vi "Serialize.vi"(0 "object in":refnum<class "Serializer.lvclass">, 2 "outputs":variant[](array[variant]), 5 "error in (no error)":errorcluster) -> (14 "object out":refnum<class "Serializer.lvclass">, 16 "JSON":string, 19 "error out":errorcluster)   [LabVIEW 2018, in "Serializer.lvclass"]
doc: "Serialize the output data to string in a format determined by the child class."
uses:
  Serializer.lvclass
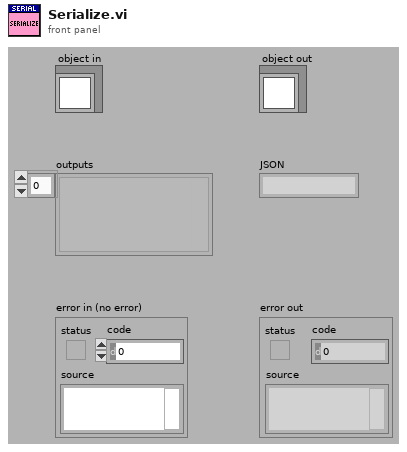
[diagram p1: front panel]
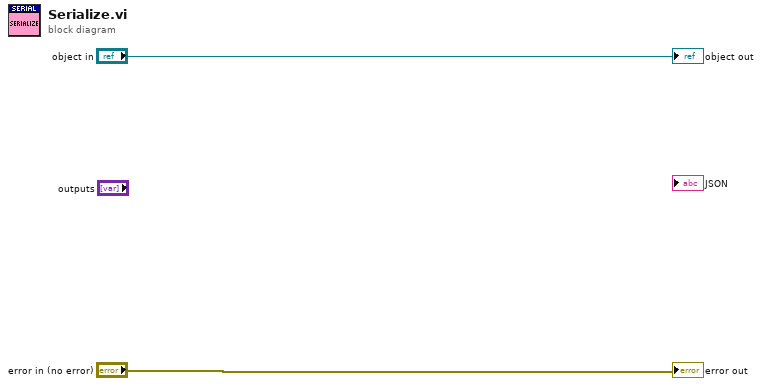
[diagram p0: block diagram]
diagram:
  "object out" <- "object in"
  "error out" <- "error in (no error)"
